vi "Get Array by name.vi"(8 "error in (no error)":errorcluster, 10 "name":string, 11 "JSON Value In":refnum<class "JSON Value.lvclass">) -> (0 "error out":errorcluster, 1 "found":bool, 2 "Array":refnum<class "JSON Value.lvclass">[](array[class]), 3 "JSON Value Out":refnum<class "JSON Value.lvclass">)   [LabVIEW 2020, in "Library Commun.lvlib" / "JSON Value.lvclass"]
doc: "Gets a <b>JSON Value</b> from a JSON collection by <b>name</b>.\n\nCopyright 2012 James David Powell, Shaun Rumbell and Ton Plomp\nMore information on http://lavag.org/topic/16217-cr-json-labview"
uses:
  JSON Value.lvclass
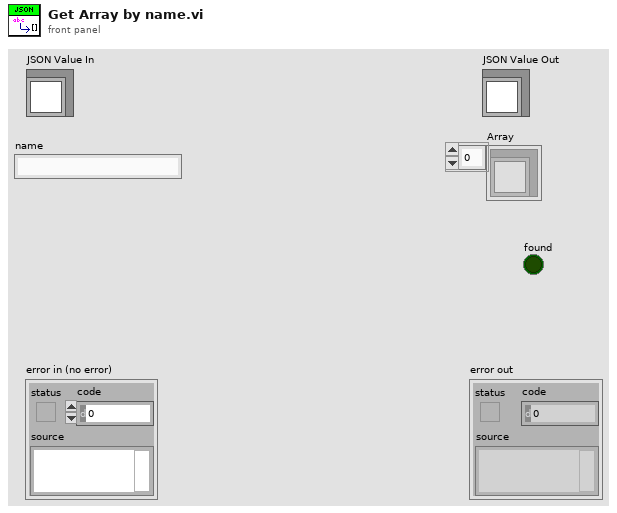
[diagram p1: front panel]
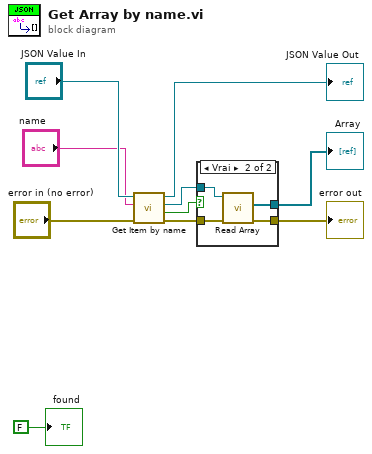
[diagram p0: block diagram]
diagram:
  n1 = call-dynamic "Get Item by name.vi"("error in (no error)"="error in (no error)", "name"="name", "JSON Value In"="JSON Value In") -> ("error out"=w1:errorcluster, "found"=w2:bool, "Value"=w3:refnum<class "JSON Value.lvclass">, "JSON Value Out"=→"JSON Value Out":refnum<class "JSON Value.lvclass">)  [unwired: 5 in]
  n2 = case shown="Vrai" w2 {
    tunnel: w3 -> [_ w15]
    tunnel: [_ w14] -> w4
    tunnel: w1 -> [w11 w13]
    tunnel: [w11 w12] -> w9
    frame False {
    }
    frame True {
      n3 = call-dynamic "Read Array.vi"("error in (no error)"=w13, "JSON Value In"=w15) -> ("error out"=w12:errorcluster, "Array"=w14:refnum<class "JSON Value.lvclass">[])  [unwired: 7 in, 1 out]
    }
  }
  "error out" <- w9
  "Array" <- w4
  "found" <- FALSE ("found")
